vi "Save_TF_Data.vi"(0 "TF_Params":T1={"Start freq (Hz)"=100.0, "Stop freq (Hz)"=50000.0, "delta f (Hz)"=100.0, "samples per channel"=100000, "fsamp (Hz)"=1000000.0, "downsampling factor"=1.0, "Attenuation factor"=1.0}, 1 "Save Raw Data?":bool, 2 "Preamp Gain":dbl=1.0, 4 "in:":path=path "D:/MPIdata", 5 "TF Mag":dbl[](array[numeric]), 6 "string":string="add_desc_here", 8 "string 2":string="TF_Tx_", 9 "TF Phase":dbl[](array[numeric]), 11 "data":dbl[][][](array[numeric]) format="%0.2f", 12 "Freqs":dbl[](array[numeric]), 13 "DividedCh2By":dbl=1.0, 14 "Output Array":dbl[](array[numeric]), 15 "DividedCh1By":dbl=1.0) -> (10 "saved name:":string="2021_08_05_15_19_22_transformer1100-50kHz_df100Hz_100kSamps_fs1M_1x_")   [LabVIEW 2021]
uses:
  <vilib>/Utility/miscctls.llb/LVRectTypeDef.ctl
  <vilib>/UPVI/lvhdf5/group.llb/H5G_obj_t.ctl
  <vilib>/UPVI/lvhdf5/dataset.llb/LVH5D Operation.ctl
  <vilib>/UPVI/lvhdf5/utility.llb/Select HDF5 Dialog.vi
  <vilib>/UPVI/lvhdf5/utility.llb/Select HDF5 Dialog (Object Only).vi
  <vilib>/UPVI/lvhdf5/dataset.llb/Simple H5Dwrite (Variant).vi
  <vilib>/UPVI/lvhdf5/attribute.llb/Write Multiple Attributes.vi
  <vilib>/UPVI/lvhdf5/attribute.llb/Simple H5Awrite (Variant).vi
  <vilib>/UPVI/lvhdf5/dataset.llb/Simple H5Dwrite.xnode
  <vilib>/UPVI/lvhdf5/library.llb/HDF5 Ref.ctl
  <vilib>/UPVI/lvhdf5/attribute.llb/LVH5A Operation.ctl
  <vilib>/UPVI/lvhdf5/attribute.llb/LVH5 Write Attributes.xnode
  <vilib>/UPVI/lvhdf5/attribute.llb/Simple H5Awrite.xnode
  <vilib>/UPVI/lvhdf5/library.llb/HDF5 Ref.lvclass
  <vilib>/UPVI/lvhdf5/identifier.llb/Not an HDF5 Refnum Constant.vi
  <vilib>/Utility/error.llb/Error Cluster From Error Code.vi
  <vilib>/UPVI/lvhdf5/dataset.llb/OpenCreateReplace Dataset by Element Type.vi
  <vilib>/UPVI/lvhdf5/dataspace.llb/H5Sselect_hyperslab.vi
  <vilib>/UPVI/lvhdf5/dataset.llb/H5Dwrite (Variant).vi
  <vilib>/UPVI/lvhdf5/dataset.llb/H5Dget_space.vi
  <vilib>/UPVI/lvhdf5/attribute.llb/private/LVH5AwriteWDTAttrs.vi
  <vilib>/UPVI/lvhdf5/dataspace.llb/H5Sclose.vi
  <vilib>/UPVI/lvhdf5/dataset.llb/H5Dclose.vi
  <vilib>/UPVI/lvhdf5/file.llb/OpenCreateReplace HDF5 File.vi
  <vilib>/UPVI/lvhdf5/file.llb/LVH5F Operation.ctl
  <vilib>/UPVI/lvhdf5/utility.llb/Select HDF5 Dialog (File and Object).vi
  <vilib>/Utility/Data Type/Get Type Information.vi
  <vilib>/Utility/Data Type/NI_Data Type.lvlib
  <vilib>/Utility/Data Type/Get Cluster Information.vi
  <vilib>/UPVI/lvhdf5/attribute.llb/Cluster to Attribute Array.xnode
panel:
  out "delta f (Hz)":dbl=25.0
  out "fsamp (Hz)":dbl=1000000.0
  out "downsampling factor":dbl=1.0
  out "Stop freq (Hz)":dbl=33000.0
  out "Start freq (Hz)":dbl=20000.0
  out "Attenuation factor":dbl=1.0
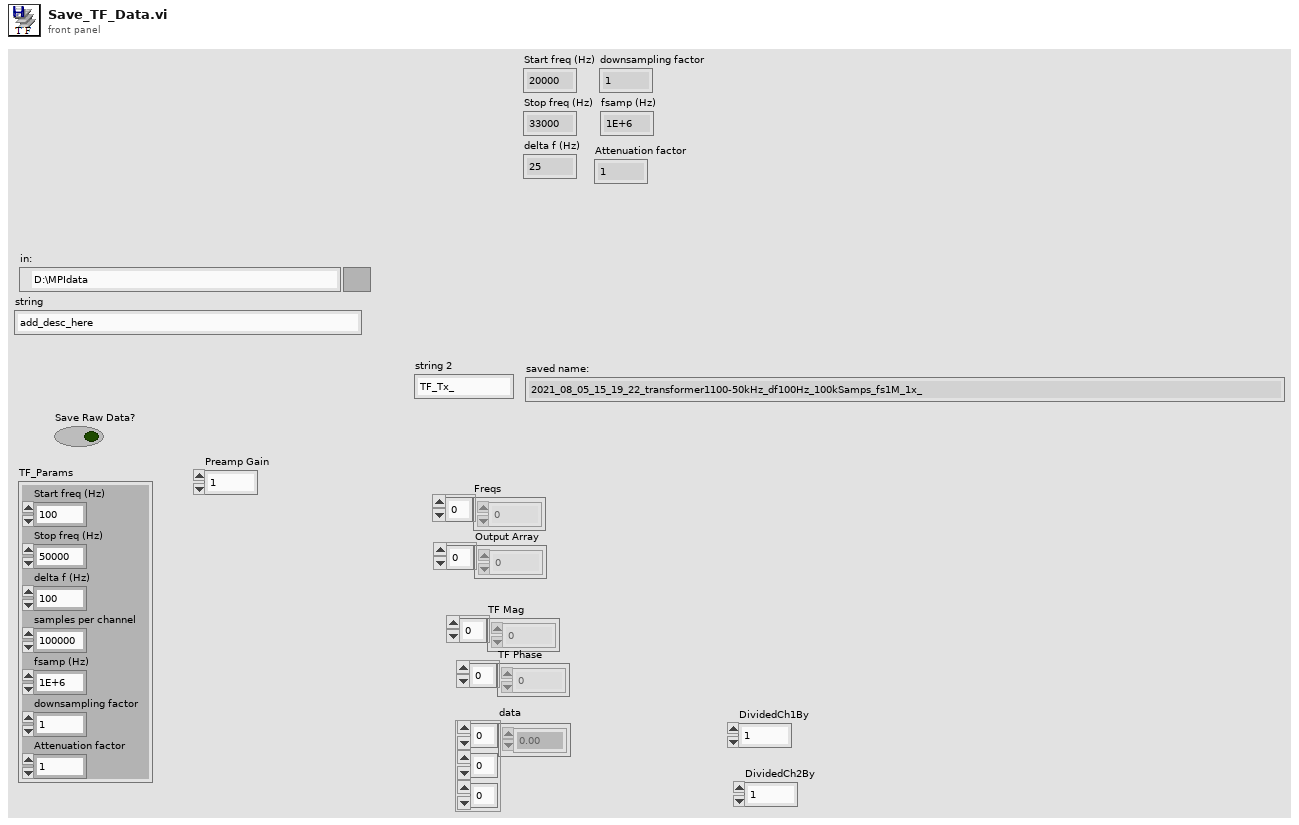
[diagram p1: front panel]
types:
  T1 = cluster{"Start freq (Hz)":dbl, "Stop freq (Hz)":dbl, "delta f (Hz)":dbl, "samples per channel":i32, "fsamp (Hz)":dbl, "downsampling factor":dbl, "Attenuation factor":dbl}
  T2 = typedef "LVRectTypeDef.ctl" = cluster{"Left":i16, "Top":i16, "Right":i16, "Bottom":i16}
  T3 = cluster{"Behavior":enum32{"Invalid", "Default", "Floating", "Floating/Auto-Hide", "Modal"}, "Position":T2, "Center":bool, "Title":string}
  T4 = typedef "LVH5F Operation.ctl" = enum16{"open", "open or create", "create or replace", "create or replace (with confirmation)", "create", "open (read only)"}
  T5 = typedef "LVH5D Operation.ctl" = enum16{"open", "replace", "create", "open or create", "create or replace", "create or replace with confirmation"}
  T6 = typedef "H5G_obj_t.ctl" = i32
  T7 = cluster{"Object Types (any)":T6[], "Object Pattern":string}
  T8 = typedef "HDF5 Ref.ctl" = refnum<class "HDF5 Ref.lvclass">
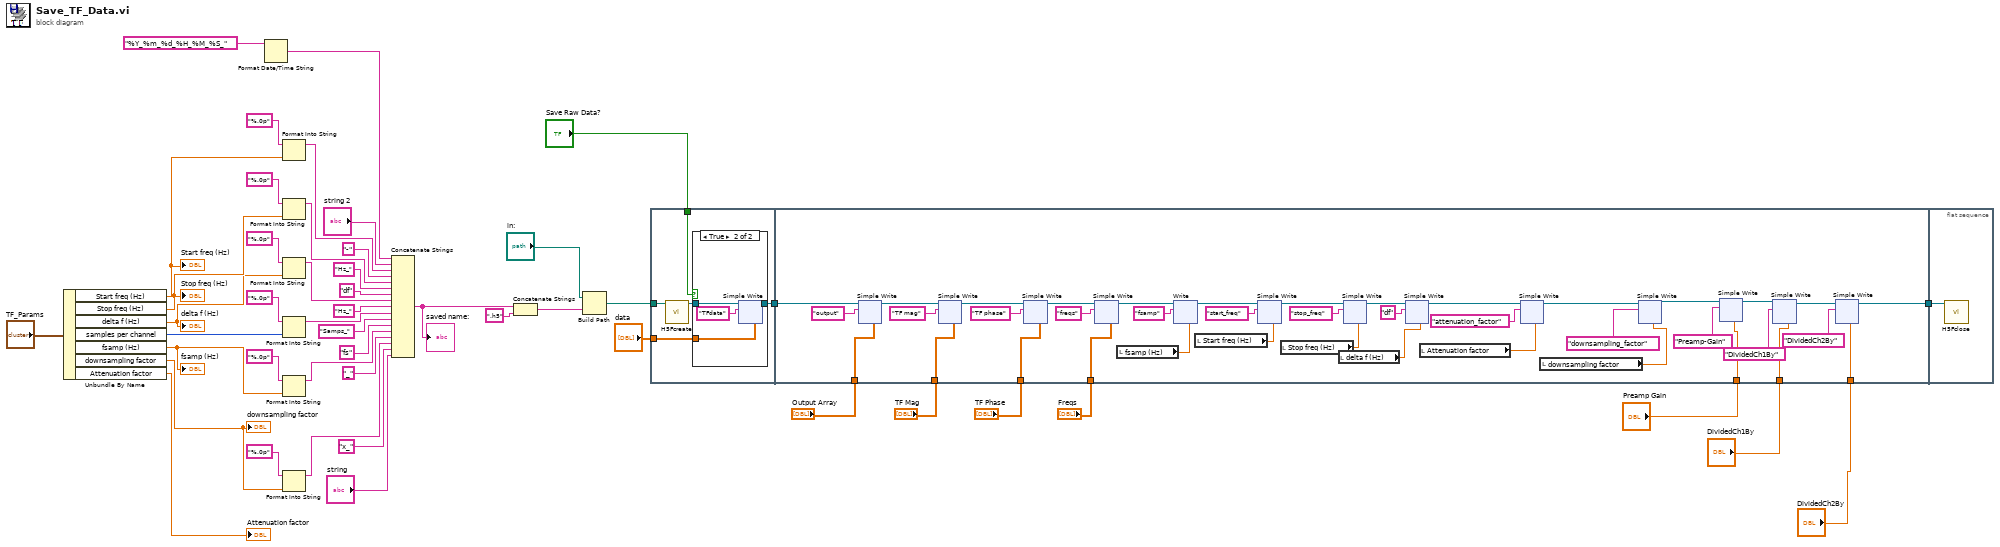
[diagram p0: block diagram]
diagram:
  n1 = Unbundle By Name("TF_Params") -> ("Start freq (Hz)"=w12:dbl, "Stop freq (Hz)"=w11:dbl, "delta f (Hz)"=w10:dbl, "samples per channel"=w9:i32, "fsamp (Hz)"=w8:dbl, "downsampling factor"=w7:dbl, "Attenuation factor"=→"Attenuation factor":dbl)
  "Start freq (Hz)" <- w12
  "Stop freq (Hz)" <- w11
  "downsampling factor" <- w7
  "fsamp (Hz)" <- w8
  "delta f (Hz)" <- w10
  n2 = Format Date/Time String(time format string (%c)="%Y_%m_%d_%H_%M_%S_") -> (date/time string=w15:string)  [unwired: 2 in]
  n3 = Format Into String(format string="%.0p", w12) -> (resulting string=w42:string)  [unwired: 2 in, 1 out]
  n4 = Format Into String(format string="%.0p", w11) -> (resulting string=w40:string)  [unwired: 2 in, 1 out]
  n5 = Format Into String(format string="%.0p", w10) -> (resulting string=w33:string)  [unwired: 2 in, 1 out]
  n6 = Format Into String(format string="%.0p", w9) -> (resulting string=w30:string)  [unwired: 2 in, 1 out]
  n7 = Format Into String(format string="%.0p", w8) -> (resulting string=w26:string)  [unwired: 2 in, 1 out]
  n8 = Format Into String(format string="%.0p", w7) -> (resulting string=w22:string)  [unwired: 2 in, 1 out]
  n9 = Concatenate Strings(w15, "string 2", w42, "-" ("string"), w40, "Hz_" ("string"), "df" ("string"), w33, "Hz_" ("string"), w30, "Samps_" ("string"), "fs" ("string"), w26, "_" ("string"), w22, "x_" ("string"), "string") -> (w28:string)
  "saved name:" <- w28
  n10 = Concatenate Strings(w28, ".h5" ("string")) -> (w45:string)
  n11 = Build Path(base path="in:", name or relative path=w45) -> (appended path=w43:path)
  n12 = flat-sequence {
    tunnel: "data" -> [w52]
    tunnel: [w51] -> w48
    tunnel: w43 -> [w50]
    tunnel: "Save Raw Data?" -> [w49]
    tunnel: [w265] -> w47
    tunnel: w48 -> [w283]
    tunnel: "Output Array" -> [w282]
    tunnel: "TF Mag" -> [w279]
    tunnel: "TF Phase" -> [w276]
    tunnel: "Freqs" -> [w271]
    tunnel: "Preamp Gain" -> [w268]
    tunnel: "DividedCh1By" -> [w262]
    tunnel: "DividedCh2By" -> [w261]
    tunnel: w47 -> [w1343]
    frame #0 {
      n13 = call <vilib>:"H5Fcreate.vi"("path"=w50) -> ("HDF5 Ref"=w53:T8)  [unwired: 7 in, 1 out]
      n14 = case shown="True" w49 {
        tunnel: w53 -> [w54 w58]
        tunnel: w52 -> [_ w56]
        tunnel: [w54 w55] -> w51
        frame False {
        }
        frame True {
          n15 = xnode "Simple Write"("Dataset Path"="TFdata", "HDF5 Path or Ref"=w58, "Data"=w56) -> ("HDF5 Ref out"=w55:T8)  [unwired: 5 in, 2 out]
        }
      }
    }
    frame #1 {
      n16 = xnode "Simple Write"("Dataset Path"="output", "HDF5 Path or Ref"=w283, "Data"=w282) -> ("HDF5 Ref out"=w280:T8)  [unwired: 5 in, 2 out]
      n17 = xnode "Simple Write"("Dataset Path"="TF mag", "HDF5 Path or Ref"=w280, "Data"=w279) -> ("HDF5 Ref out"=w277:T8)  [unwired: 5 in, 2 out]
      n18 = xnode "Simple Write"("Dataset Path"="TF phase", "HDF5 Path or Ref"=w277, "Data"=w276) -> ("HDF5 Ref out"=w274:T8)  [unwired: 5 in, 2 out]
      n19 = xnode "Simple Write"("Dataset Path"="freqs", "HDF5 Path or Ref"=w274, "Data"=w271) -> ("HDF5 Ref out"=w273:T8)  [unwired: 5 in, 2 out]
      n20 = local read "fsamp (Hz)"() -> (w299:dbl)
      n21 = xnode "Write"("HDF5 Ref"=w273, "Name(s)"="fsamp", "Value(s)"=w299) -> ("HDF5 Ref out"=w296:T8)  [unwired: 2 in, 1 out]
      n22 = local read "Start freq (Hz)"() -> (w294:dbl)
      n23 = xnode "Simple Write"("HDF5 Ref"=w296, "Name"="start_freq", "Value"=w294) -> ("HDF5 Ref out"=w293:T8)  [unwired: 2 in, 1 out]
      n24 = local read "Stop freq (Hz)"() -> (w291:dbl)
      n25 = local read "delta f (Hz)"() -> (w297:dbl)
      n26 = xnode "Simple Write"("HDF5 Ref"=w293, "Name"="stop_freq", "Value"=w291) -> ("HDF5 Ref out"=w292:T8)  [unwired: 2 in, 1 out]
      n27 = xnode "Simple Write"("HDF5 Ref"=w292, "Name"="df", "Value"=w297) -> ("HDF5 Ref out"=w289:T8)  [unwired: 2 in, 1 out]
      n28 = local read "Attenuation factor"() -> (w285:dbl)
      n29 = xnode "Simple Write"("HDF5 Ref"=w289, "Name"="attenuation_factor", "Value"=w285) -> ("HDF5 Ref out"=w288:T8)  [unwired: 2 in, 1 out]
      n30 = local read "downsampling factor"() -> (w284:dbl)
      n31 = xnode "Simple Write"("HDF5 Ref"=w288, "Name"="downsampling_factor", "Value"=w284) -> ("HDF5 Ref out"=w270:T8)  [unwired: 2 in, 1 out]
      n32 = xnode "Simple Write"("HDF5 Ref"=w270, "Name"="Preamp-Gain", "Value"=w268) -> ("HDF5 Ref out"=w267:T8)  [unwired: 2 in, 1 out]
      n33 = xnode "Simple Write"("HDF5 Ref"=w267, "Name"="DividedCh1By", "Value"=w262) -> ("HDF5 Ref out"=w266:T8)  [unwired: 2 in, 1 out]
      n34 = xnode "Simple Write"("HDF5 Ref"=w266, "Name"="DividedCh2By", "Value"=w261) -> ("HDF5 Ref out"=w265:T8)  [unwired: 2 in, 1 out]
    }
    frame #2 {
      n35 = call <vilib>:"H5Fclose.vi"("HDF5 Ref"=w1343) -> ()  [unwired: 8 in, 1 out]
    }
  }
